vi "TestMan-Complex example.vi"() -> ()   [LabVIEW 2013]
uses:
  <vilib>/Platform/storage/lvStorage.llb/_openFunction.ctl
  builds/udp_example/udp/udp.lvlibp/serverID.vi
  <vilib>/Platform/storage/lvStorage.llb/_openStorageWithRootAutoDetect.vi
  <vilib>/Platform/storage/lvStorage.llb/xStorage/xStorageSupp/ErrorOut.vi
  <vilib>/Platform/storage/lvStorage.llb/_queryPropPoly.vi
  <vilib>/Platform/storage/lvStorage.llb/_queryPropString.vi
  <vilib>/Platform/storage/lvStorage.llb/_queryGenericObjects.vi
  <vilib>/Platform/storage/lvStorage.llb/_loadAllDouble.vi
  <vilib>/Platform/storage/Storage.llb/Get Object Info.vi
  <vilib>/Platform/storage/Storage.llb/__closeStorageFromObject.vi
  <vilib>/measure/maspectr.llb/FFT Power Spectrum for 1 Chan.vi
  <vilib>/Platform/storage/lvStorage.llb/xStorage/Open Data Storage/Open Data Storage.xnode
  <vilib>/Platform/storage/lvStorage.llb/xStorage/Read Data/Read Data.xnode
  <vilib>/Platform/storage/lvStorage.llb/xStorage/Close Data Storage/Close Data Storage.xnode
  builds/udp_example/udp/udp.lvlibp
  <vilib>/measure/NI_MAPro.lvlib
panel:
  out "Spectrum":cluster{dbl[], "magnitude":dbl[]}(graph)
  out "Command?":bool
  out "TX data":cdb[](array[numeric])
  in  "TX Gain [dB]":dbl=30.0 format="%#_6f"
  in  "TX IQ rate":dbl=1000000.0 format="%#_6p"
  in  "TX data":path
  out "curent state":enum16{"Wait", "Configure", "Run", "Stop"}(ring)
  out "error out":errorcluster
  out "Received Packet":string="New TX data received"
  in  "RX IQ Sampling\nRate [S/sec]":dbl=1000000.0 format="%#.6p"
  in  "Carrier\nFrequency [Hz]":dbl=1990000000.0 format="%#.6p"
  in  "RX Gain [dB]":dbl=29.0 format="%#.6p"
  in  "Run TX":bool
  in  "ipadress":string="224.5.6.7"
  in  "port":i32=50000
  in  "ttl":i32=1
  in  "type TX":u8=150
  in  "id":u8=100
  in  "Configure UDP":bool
  in  "stop":bool
  # "Application Configuration"
  # "USRP Configuration"
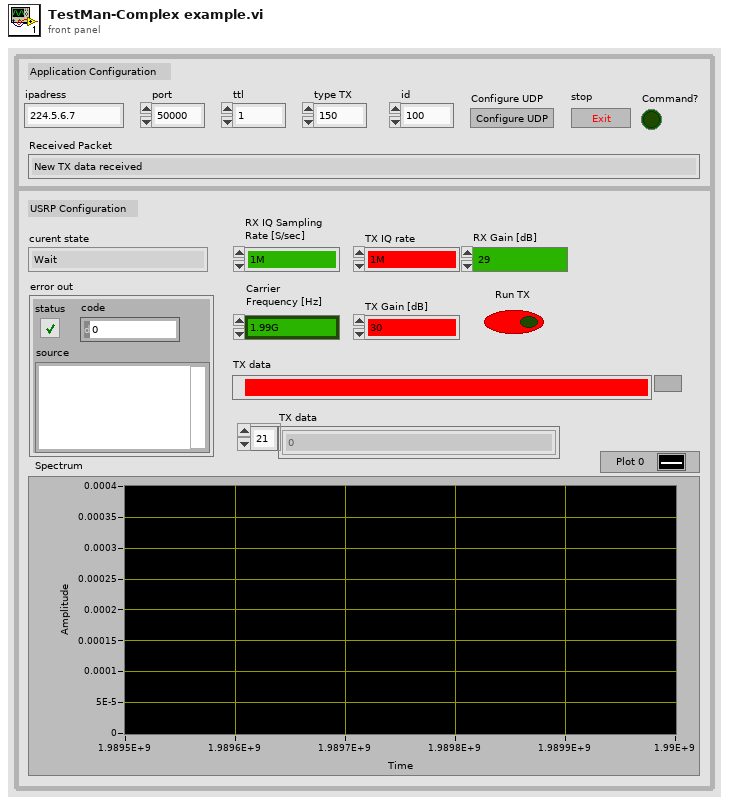
[diagram p1: front panel]
types:
  T1 = enum8{"Enabled", "Disabled", "Disabled and Grayed Out"}
  T2 = enum16{"UPDATE", "READ", "QUERY", "CREATE CHILD", "CREATE", "CONNECT", "DISCONNECT"}
  T3 = typedef "_openFunction.ctl" = enum16{"open", "open or create", "create or replace", "create", "open (read only)"}
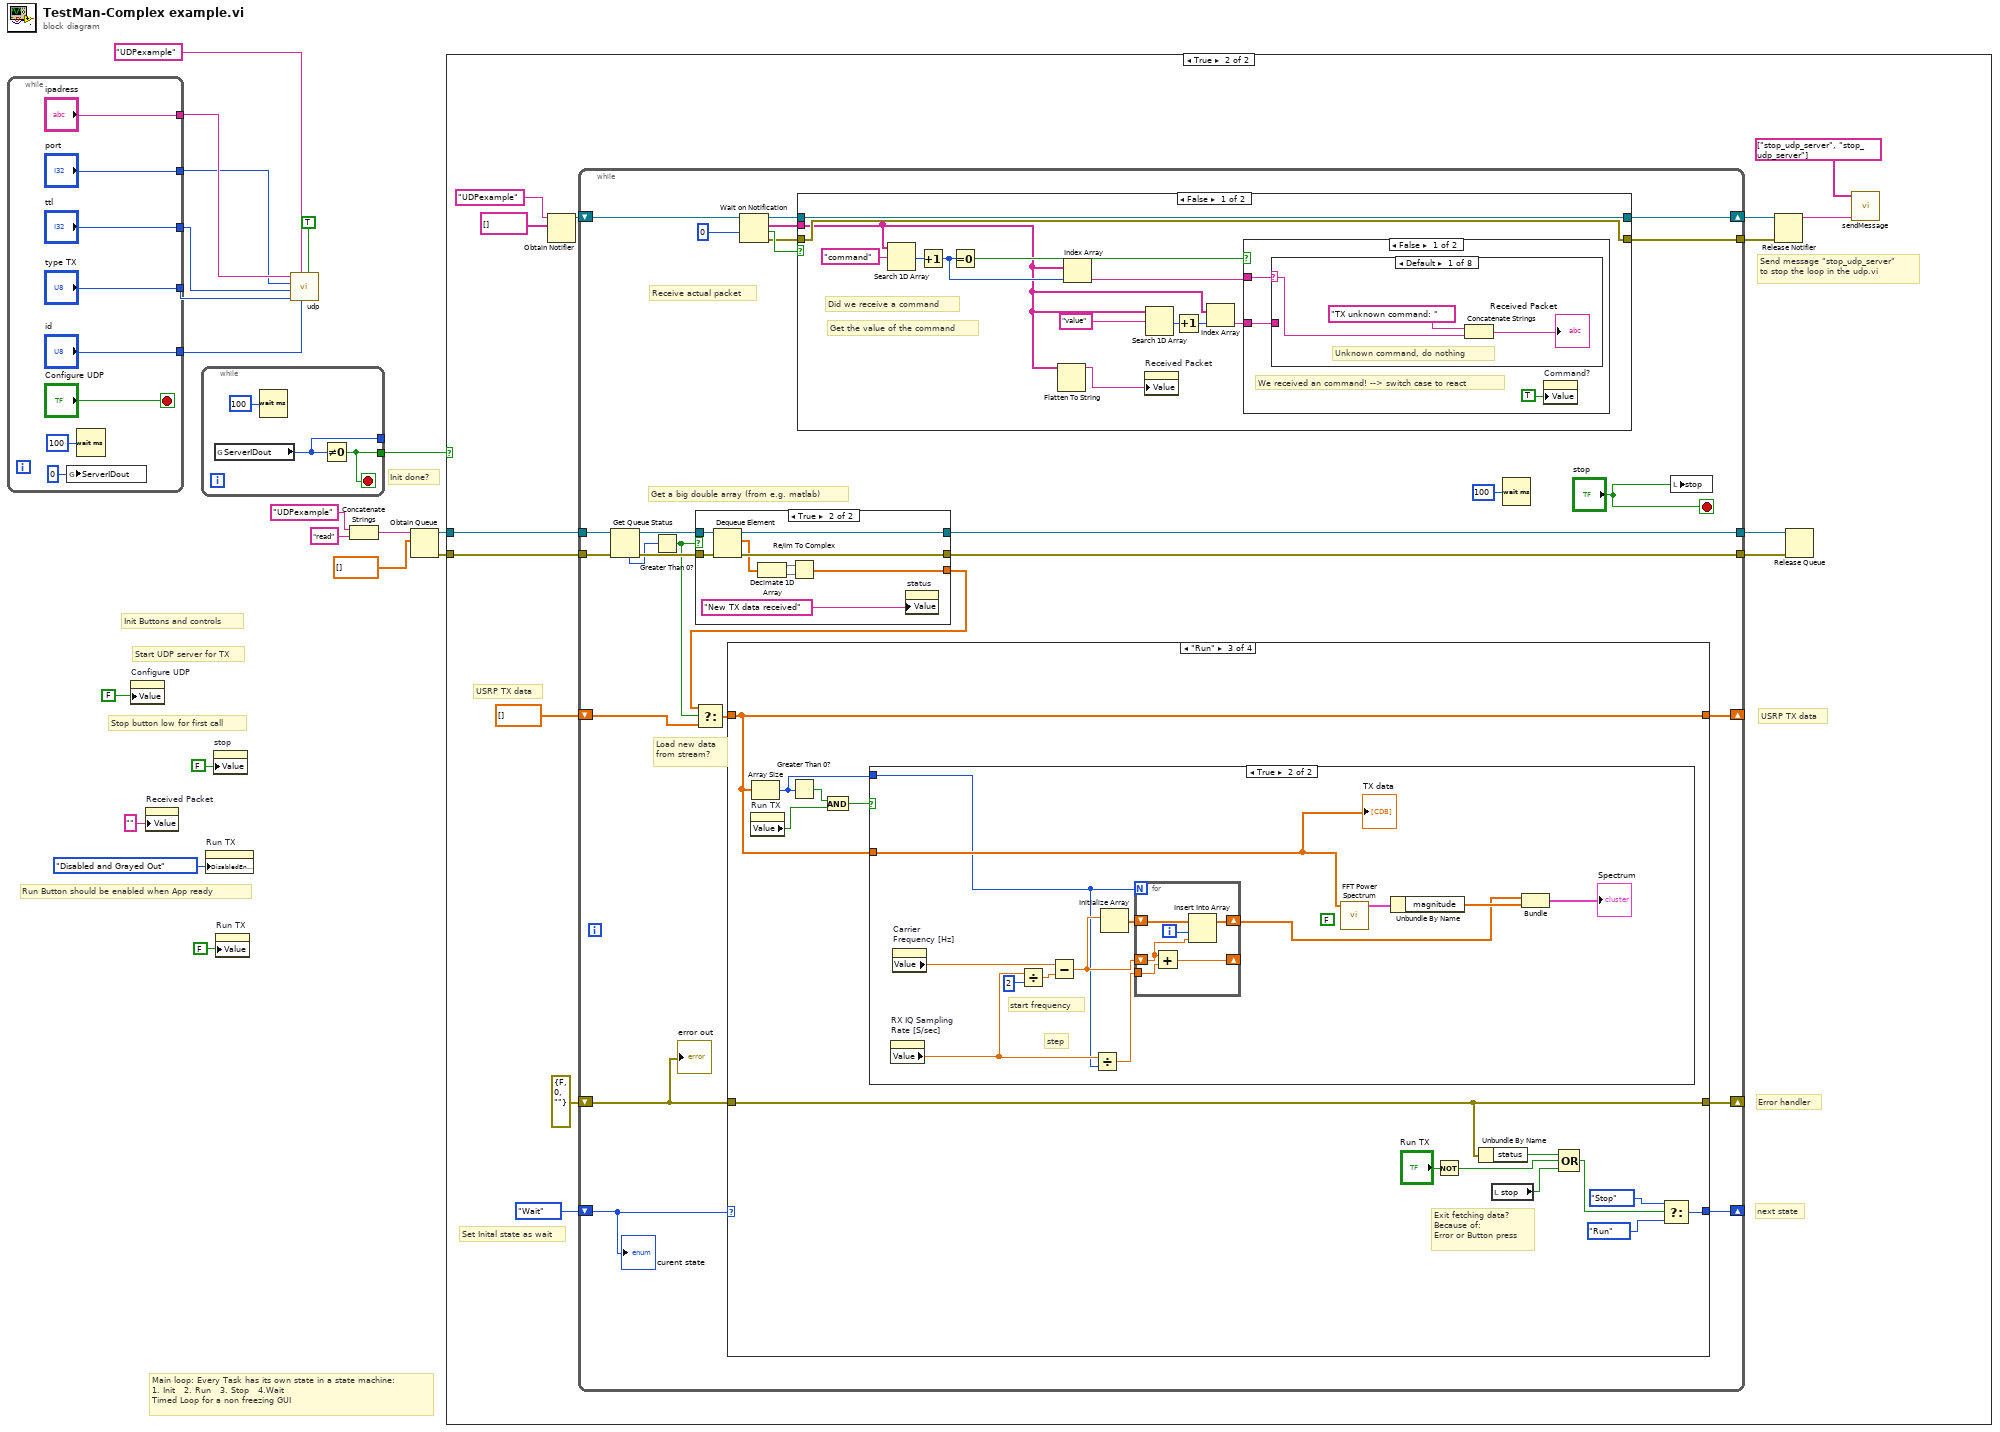
[diagram p0: block diagram]
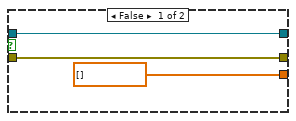
[diagram p3: hidden frame]
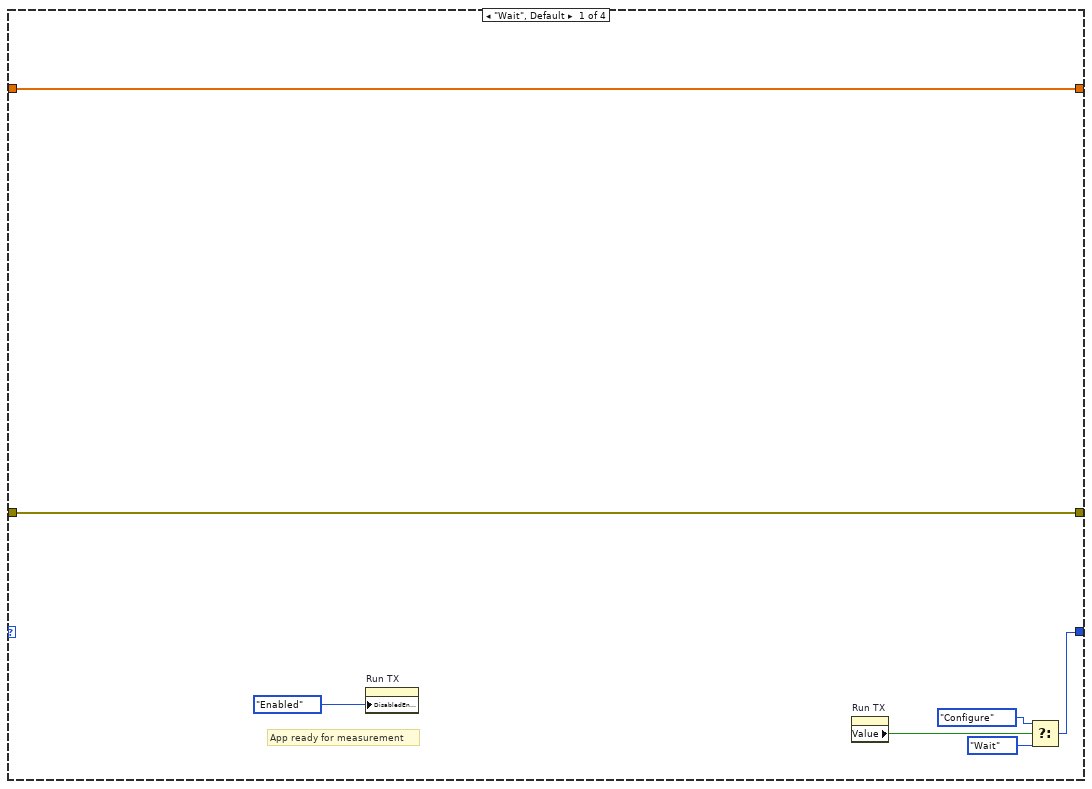
[diagram p4: hidden frame]
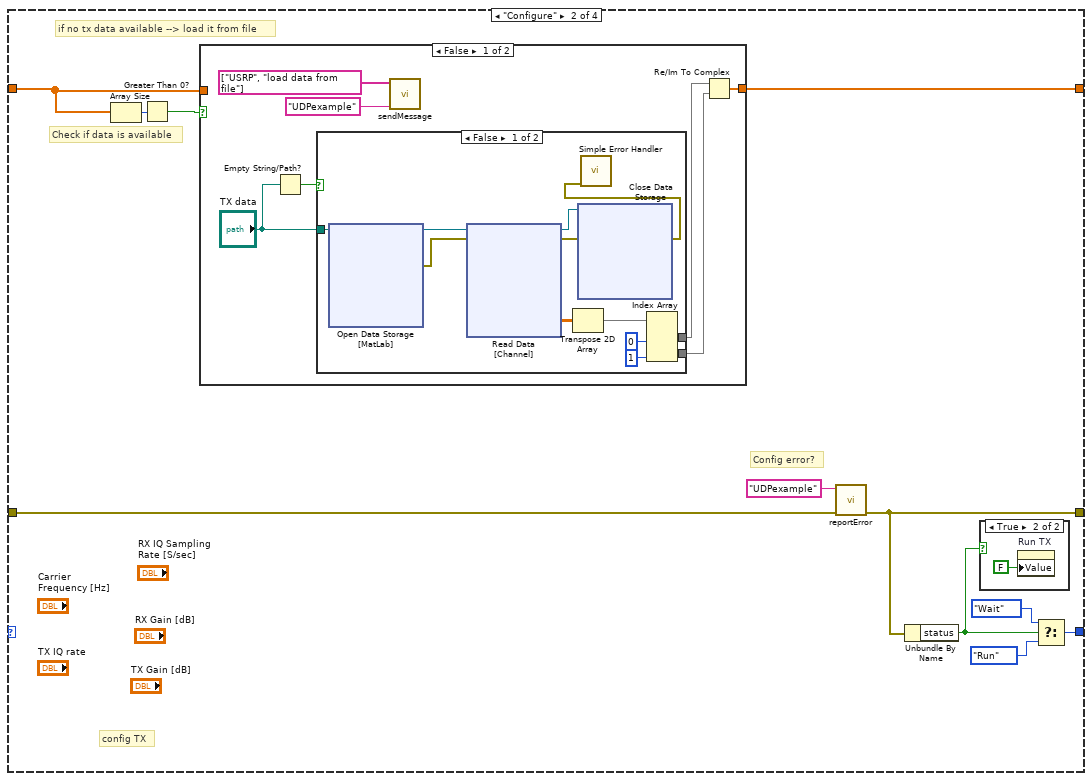
[diagram p5: hidden frame]
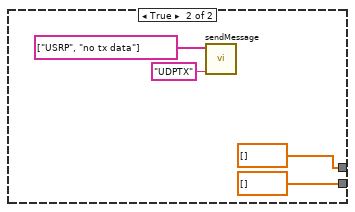
[diagram p6: hidden frame]
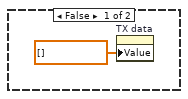
[diagram p9: hidden frame]
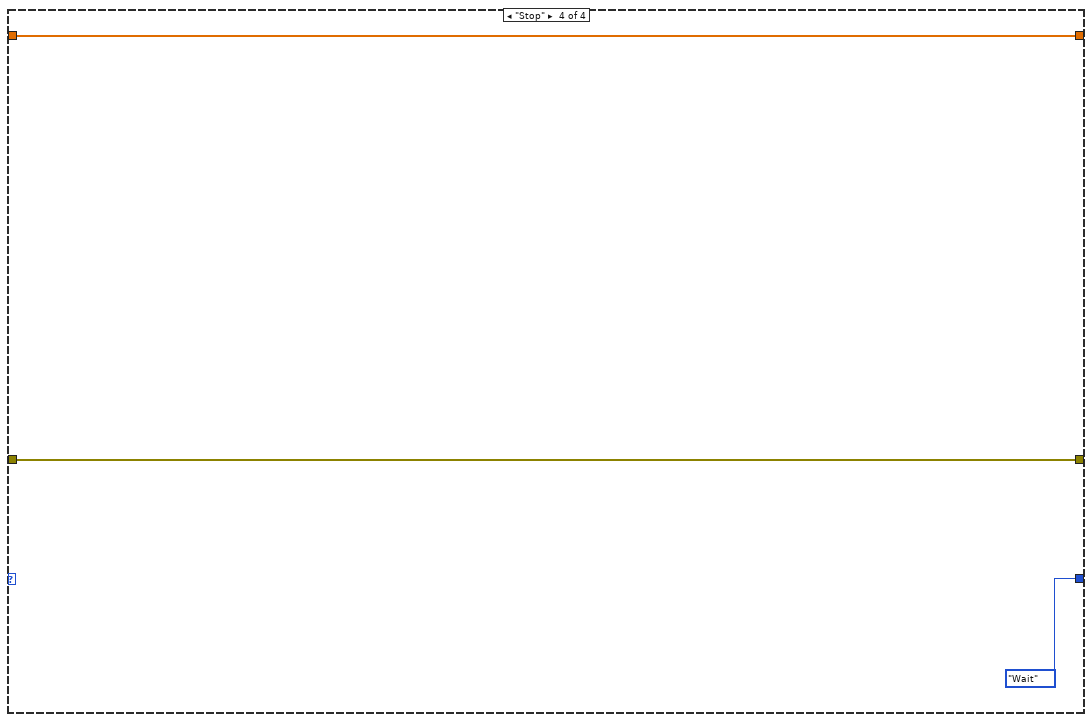
[diagram p10: hidden frame]
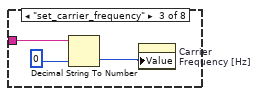
[diagram p12: hidden frame]
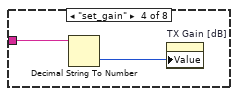
[diagram p13: hidden frame]
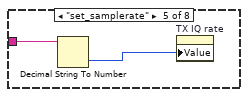
[diagram p14: hidden frame]
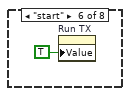
[diagram p15: hidden frame]
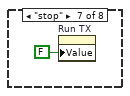
[diagram p16: hidden frame]
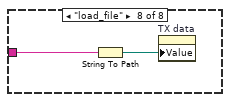
[diagram p17: hidden frame]
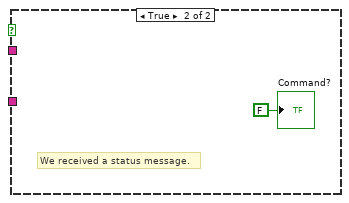
[diagram p18: hidden frame]
diagram:
  # "Init Buttons and controls"
  # "Start UDP server for TX"
  # "Main loop: Every Task has its own state in a state machine:\n1. Init   2. Run   3. Stop   4.Wait\nTimed Loop for a non freezing GUI"
  # "Run Button should be enabled when App ready"
  # "Init done?"
  # "Stop button low for first call"
  n1 = while {
    tunnel: ["ipadress"] -> w12
    tunnel: ["port"] -> w11
    tunnel: ["ttl"] -> w10
    tunnel: ["type TX"] -> w13
    tunnel: ["id"] -> w19
    stop <- "Configure UDP" stop-if-true
    n2 = global write "serverID.vi" "ServerIDout"(u8 0 ("ServerIDout")) -> ()
    n3 = Wait (ms)(milliseconds to wait=u32 100) -> ()  [unwired: 1 out]
  }
  n4 = property on="Configure UDP" class="Bool (strict)"("Value"=FALSE ("stop")) -> ()  [unwired: 2 in, 2 out]
  n5 = property on="Received Packet" class="Str"("Value"="" ("Received Command")) -> ()  [unwired: 2 in, 2 out]
  n6 = while {
    tunnel: [w29] -> w9
    tunnel: [w28] -> _
    stop <- w29 stop-if-true
    n7 = global read "serverID.vi" "ServerIDout"() -> (w28:u8)
    n8 = Wait (ms)(milliseconds to wait=u32 100) -> ()  [unwired: 1 out]
    n9 = Not Equal To 0?(x=w28) -> (x != 0?=w29:bool)
  }
  n10 = property on="Run TX" class="Bool (strict)"("DisabledEnum"=T1."Disabled and Grayed Out" ("Disabled")) -> ()  [unwired: 2 in, 2 out]
  n11 = property on="stop" class="Bool (strict)"("Value"=FALSE ("stop")) -> ()  [unwired: 2 in, 2 out]
  n12 = property on="Run TX" class="Bool (strict)"("Value"=FALSE ("Run")) -> ()  [unwired: 2 in, 2 out]
  n13 = call "udp.vi"("Get stream data as doubles"=TRUE, "id in"=w19, "name"="UDPexample", "type in"=w13, "ttl in"=w10, "port in"=w11, "ipadress in"=w12) -> ()  [unwired: 2 in, 2 out]
  n14 = Concatenate Strings("UDPexample" ("name"), "read" ("string")) -> (w7:string)
  n15 = Obtain Queue(name (unnamed)=w7, element data type=dbl[] [] ("GetDoubles")) -> (queue out=w3:refnum<queue>, error out=w2:errorcluster)  [unwired: 3 in, 1 out]
  n16 = case shown="True" w9 {
    tunnel: w3 -> [_ w36]
    tunnel: w2 -> [_ w35]
    frame False {
    }
    frame True {
      # "Send message \"stop_udp_server\"\nto stop the loop in the udp.vi"
      # "next state"
      # "USRP TX data"
      # "USRP TX data"
      # "Set Inital state as wait"
      # "Error handler"
      n17 = Obtain Notifier(name (unnamed)="UDPexample" ("name"), notification data type=string[] []) -> (notifier out=w44:refnum<notifier>)  [unwired: 2 in, 2 out]
      n18 = while {
        shift-right: [w70] -> w43
        shift-left: w44 -> [w68]
        shift-right: [w62] -> _
        shift-left: enum16{"Wait", "Configure", "Run", "Stop"}."Wait" -> [w63]
        shift-right: [w61] -> _
        shift-left: errorcluster {"status"=FALSE, "code"=0, "source"=""} ("error out") -> [w60]
        shift-right: [w59] -> _
        shift-left: dbl[] [] -> [w57]
        tunnel: w36 -> [w53]
        tunnel: w35 -> [w52]
        tunnel: [w51] -> w34
        tunnel: [w50] -> w33
        tunnel: [w46] -> w32
        stop <- "stop" stop-if-true
        # "Load new data\nfrom stream?"
        # "Get a big double array (from e.g. matlab)"
        # "Receive actual packet"
        n19 = Get Queue Status(queue=w53, error in (no error)=w52) -> (queue out=w56:refnum<queue>, error out=w55:errorcluster, # elements in queue=w54:i32)  [unwired: 1 in, 5 out]
        n20 = Greater Than 0?(x=w54) -> (x > 0?=w49:bool)
        n21 = case shown="True" w49 {
          tunnel: w56 -> [w73 w82]
          tunnel: w55 -> [w72 w81]
          tunnel: [w73 w80] -> w51
          tunnel: [w72 w79] -> w50
          tunnel: [cdb[] [] w75] -> w48
          frame False {
          }
          frame True {
            n22 = Dequeue Element(queue=w82, error in (no error)=w81) -> (queue out=w80:refnum<queue>, element=w76:dbl[], error out=w79:errorcluster)  [unwired: 1 in, 1 out]
            n23 = Decimate 1D Array(w76) -> (w78:dbl[], w77:dbl[])
            n24 = Re/Im To Complex(1:w77, 2:w78) -> (0:w75:cdb[])
            n25 = property on="status" class="Str"("Value"="New TX data received" ("Received Command")) -> ()  [unwired: 2 in, 2 out]
          }
        }
        n26 = Select(t=w48, s=w49, f=w57) -> (s? t:f=w58:cdb[])
        n27 = case shown="\"Run\"" w63 {
          tunnel: [w87 w100 w169 enum16{"Wait", "Configure", "Run", "Stop"}."Wait"] -> w62
          tunnel: [w84 w91 w164 w194] -> w61
          tunnel: w60 -> [w84 w90 w164 w194]
          tunnel: w58 -> [w88 w93 w163 w195]
          tunnel: [w88 w94 w163 w195] -> w59
          frame "Wait", Default {
            # "App ready for measurement"
            n28 = property on="Run TX" class="Bool (strict)"("DisabledEnum"=T1."Enabled" ("Disabled")) -> ()  [unwired: 2 in, 2 out]
            n29 = property on="Run TX" class="Bool (strict)"() -> ("Value"=w83:bool)  [unwired: 2 in, 2 out]
            n30 = Select(t=enum16{"Wait", "Configure", "Run", "Stop"}."Configure", s=w83, f=enum16{"Wait", "Configure", "Run", "Stop"}."Wait") -> (s? t:f=w87:enum16{"Wait", "Configure", "Run", "Stop"})
          }
          frame "Configure" {
            # "config TX"
            # "Config error?"
            # "if no tx data available --> load it from file"
            # "Check if data is available"
            n31 = Array Size(array=w93) -> (size(s)=w96:i32)
            n32 = Greater Than 0?(x=w96) -> (x > 0?=w95:bool)
            n33 = case shown="False" w95 {
              tunnel: [w102 w158] -> w94
              tunnel: w93 -> [_ w158]
              frame False {
                n34 = Empty String/Path?(string/path="TX data") -> (empty?=w106:bool)
                n35 = case shown="False" w106 {
                  tunnel: [w110 dbl[] []] -> w104
                  tunnel: [w109 dbl[] []] -> w103
                  tunnel: "TX data" -> [w108 _]
                  frame False {
                    n36 = xnode "Open Data Storage\n[MatLab]"("file path"=w108) -> ("storage refnum (file)"=w119:refnum<k20>, "error out"=w113:errorcluster)  [unwired: 4 in, 1 out]
                    n37 = xnode "Read Data\n[Channel]"("storage refnum (file)"=w119, "error in"=w113) -> ("Signal"=w116:dbl[][], "storage refnum (file) out"=w114:refnum<k20>, "error out"=w112:errorcluster)  [unwired: 2 in, 1 out]
                    n38 = Transpose 2D Array(2D array=w116) -> (transposed array=w115:dbl[][])
                    n39 = xnode "Close Data Storage\n"("storage refnum (file)"=w114, "error in (no error)"=w112) -> ("error out"=w111:errorcluster)  [unwired: 1 out]
                    n40 = call <vilib>:"Simple Error Handler.vi"("error in (no error)"=w111) -> ()  [unwired: 4 in, 5 out]
                    n41 = Index Array(array=w115, index (col) #1=0 ("disabled index (col)"), index (col) #2=1 ("index (col)")) -> (element #1=w110:dbl[], element #2=w109:dbl[])  [unwired: 2 in]
                  }
                  frame True {
                    n42 = call "sendMessage.vi"("name (UDP)"="UDPTX", "message"=string[] ["USRP", "no tx data"]) -> ()  [unwired: 10 in]
                  }
                }
                n43 = call "sendMessage.vi"("name (UDP)"="UDPexample", "message"=string[] ["USRP", "load data from file"]) -> ()  [unwired: 10 in]
                n44 = Re/Im To Complex(1:w103, 2:w104) -> (0:w102:cdb[])
              }
              frame True {
              }
            }
            n45 = call "reportError.vi"("error in (no error)"=w90, "name (UDP)"="UDPexample") -> ("error out"=w91:errorcluster)  [unwired: 9 in]
            n46 = Unbundle By Name(w91) -> ("status"=w97:bool)
            n47 = case shown="True" w97 {
              frame False {
              }
              frame True {
                n48 = property on="Run TX" class="Bool (strict)"("Value"=FALSE ("Run")) -> ()  [unwired: 2 in, 2 out]
              }
            }
            n49 = Select(t=enum16{"Wait", "Configure", "Run", "Stop"}."Wait", s=w97, f=enum16{"Wait", "Configure", "Run", "Stop"}."Run") -> (s? t:f=w100:enum16{"Wait", "Configure", "Run", "Stop"})
          }
          frame "Run" {
            # "Exit fetching data?\nBecause of:\nError or Button press"
            n50 = property on="Run TX" class="Bool (strict)"() -> ("Value"=w165:bool)  [unwired: 2 in, 2 out]
            n51 = Array Size(array=w163) -> (size(s)=w162:i32)
            n52 = Greater Than 0?(x=w162) -> (x > 0?=w166:bool)
            n53 = And(x=w166, y=w165) -> (x .and. y?=w167:bool)
            n54 = case shown="True" w167 {
              tunnel: w163 -> [_ w185]
              tunnel: w162 -> [_ w177]
              frame False {
                n55 = property on="TX data" class="Arr (strict)"("Value"=cdb[] [] ("TX data")) -> ()  [unwired: 2 in, 2 out]
              }
              frame True {
                (unwired) FALSE ("dB On (F)")
                # "step"
                # "start frequency"
                n56 = property on="RX IQ Sampling\nRate [S/sec]" class="DigNum (strict)"() -> ("Value"=w178:dbl)  [unwired: 2 in, 2 out]
                n57 = property on="Carrier\nFrequency [Hz]" class="DigNum (strict)"() -> ("Value"=w179:dbl)  [unwired: 2 in, 2 out]
                n58 = Divide(x=w178, y=u8 2) -> (x/y=w184:dbl)
                n59 = Subtract(x=w179, y=w184) -> (x-y=w181:dbl)
                n60 = Divide(x=w178, y=w177) -> (x/y=w180:dbl)
                n61 = Initialize Array(w181) -> (w182:dbl[])  [unwired: 1 in]
                n62 = for {
                  N: w177 -> [_]
                  shift-right: [w193] -> w176
                  shift-left: w182 -> [w192]
                  shift-right: [w190] -> _
                  shift-left: w181 -> [w188]
                  tunnel: w180 -> [w189]
                  i -> [w191]
                  n63 = Add(x=w188, y=w189) -> (x+y=w190:dbl)
                  n64 = Insert Into Array(array=w192, index=w191, new element=w188) -> (w193:dbl[])
                }
                n65 = call-poly <vilib>:"FFT Power Spectrum.vi"("time signal"=w185) -> ("power spectrum"=w186:cluster{"f0":dbl, "df":dbl, "magnitude":dbl[]})  [unwired: 7 in, 3 out]
                n66 = Unbundle By Name(w186) -> ("magnitude"=w187:dbl[])
                n67 = Bundle(w176, "magnitude"=w187) -> (→"Spectrum":cluster{dbl[], "magnitude":dbl[]})  [unwired: 1 in]
                "TX data" <- w185
              }
            }
            n68 = Not(x="Run TX") -> (.not. x?=w160:bool)
            n69 = Unbundle By Name(w164) -> ("status"=w173:bool)
            n70 = local read "stop"() -> (w168:bool)
            n71 = Compound Arithmetic op=OR(w173, w160, w168) -> (w172:bool)
            n72 = Select(t=enum16{"Wait", "Configure", "Run", "Stop"}."Stop", s=w172, f=enum16{"Wait", "Configure", "Run", "Stop"}."Run") -> (s? t:f=w169:enum16{"Wait", "Configure", "Run", "Stop"})
          }
          frame "Stop" {
          }
        }
        n73 = Wait on Notification(notifier=w68, timeout in ms (-1)=0) -> (notifier out=w67:refnum<notifier>, notification=w64:string[], timed out?=w66:bool, error out=w45:errorcluster)  [unwired: 2 in]
        n74 = case shown="False" w66 {
          tunnel: [w209 w229] -> w70
          tunnel: w67 -> [w209 w229]
          tunnel: w64 -> [w197 _]
          tunnel: [w199 w228] -> w46
          tunnel: w45 -> [w199 w228]
          frame False {
            # "Get the value of the command"
            # "Did we receive a command"
            n75 = Search 1D Array(1D array=w197, element="command") -> (index of element=w207:i32)  [unwired: 1 in]
            n76 = Increment(x=w207) -> (x+1=w205:i32)
            n77 = Equal To 0?(x=w205) -> (x = 0?=w206:bool)
            n78 = Flatten To String(anything=w197) -> (data string=w198:string)  [unwired: 3 in, 2 out]
            n79 = Index Array(array=w197, index=w205) -> (element=w204:string)
            n80 = property on="Received Packet" class="Str"("Value"=w198) -> ()  [unwired: 2 in, 2 out]
            n81 = Search 1D Array(1D array=w197, element="value") -> (index of element=w200:i32)  [unwired: 1 in]
            n82 = Increment(x=w200) -> (x+1=w201:i32)
            n83 = Index Array(array=w197, index=w201) -> (element=w202:string)
            n84 = case shown="False" w206 {
              tunnel: w204 -> [w212 _]
              tunnel: w202 -> [w211 _]
              frame False {
                # "We received an command! --> switch case to react"
                n85 = case shown="Default" w212 {
                  selector: w212 -> [w214 _ _ _ _ _ _ _]
                  tunnel: w211 -> [_ _ w218 w220 w222 _ _ w226]
                  frame Default {
                    # "Unknown command, do nothing"
                    n86 = Concatenate Strings("TX unknown command: " ("string"), w214) -> (→"Received Packet":string)
                  }
                  frame "set_usrp_ipaddress" {
                  }
                  frame "set_carrier_frequency" {
                    n87 = Decimal String To Number(string=w218, default (0L)=u64 0) -> (number=w217:u64)  [unwired: 1 in, 1 out]
                    n88 = property on="Carrier\nFrequency [Hz]" class="DigNum (strict)"("Value"=w217) -> ()  [unwired: 2 in, 2 out]
                  }
                  frame "set_gain" {
                    n89 = Decimal String To Number(string=w220) -> (number=w219:i32)  [unwired: 2 in, 1 out]
                    n90 = property on="TX Gain [dB]" class="DigNum (strict)"("Value"=w219) -> ()  [unwired: 2 in, 2 out]
                  }
                  frame "set_samplerate" {
                    n91 = Decimal String To Number(string=w222) -> (number=w221:i32)  [unwired: 2 in, 1 out]
                    n92 = property on="TX IQ rate" class="DigNum (strict)"("Value"=w221) -> ()  [unwired: 2 in, 2 out]
                  }
                  frame "start" {
                    n93 = property on="Run TX" class="Bool (strict)"("Value"=TRUE ("Run")) -> ()  [unwired: 2 in, 2 out]
                  }
                  frame "stop" {
                    n94 = property on="Run TX" class="Bool (strict)"("Value"=FALSE ("Run")) -> ()  [unwired: 2 in, 2 out]
                  }
                  frame "load_file" {
                    n95 = String To Path(string=w226) -> (path=w225:path)
                    n96 = property on="TX data" class="Path"("Value"=w225) -> ()  [unwired: 2 in, 2 out]
                  }
                }
                n97 = property on="Command?" class="Bool (strict)"("Value"=TRUE ("Command?")) -> ()  [unwired: 2 in, 2 out]
              }
              frame True {
                # "We received a status message."
                "Command?" <- FALSE ("Command?")
              }
            }
          }
          frame True {
          }
        }
        n98 = Wait (ms)(milliseconds to wait=u32 100) -> ()  [unwired: 1 out]
        n99 = local write "stop"("stop") -> ()
        "error out" <- w60
        "curent state" <- w63
      }
      n100 = Release Notifier(notifier=w43, error in (no error)=w32) -> (notifier name=w39:string)  [unwired: 1 in, 2 out]
      n101 = Release Queue(queue=w34, error in (no error)=w33) -> ()  [unwired: 1 in, 3 out]
      n102 = call "sendMessage.vi"("name (UDP)"=w39, "message"=string[] ["stop_udp_server", "stop_udp_server"]) -> ()  [unwired: 10 in]
    }
  }
